vi "Generic command handler.vi"(8 "error in (no error)":errorcluster, 10 "Message in":refnum<class "GenericMessage.lvclass">=refnum, 11 "PockelCell in":refnum<class "PockelCell.lvclass">) -> (0 "error out":errorcluster, 2 "value":string, 3 "PockelCell out":refnum<class "PockelCell.lvclass">)   [LabVIEW 2012, in "PockelCell.lvclass"]
doc: "The generic_command_handler processes the command 'generic'. Commands which are not part of the predefined list of commands fall under the 'generic' command for special activity."
uses:
  PockelCell.lvclass
  <vilib>/Distrio/Murmex/Murmex/Murmex.lvclass
  Murmex/LabVIEW/Murmex/GenericMessage/GenericMessage.lvclass
panel:
  # "This method is called when the GENERIC\ntrigger is sent. \n\nOverride this method when your component needs to\nrespond to this trigger. \n\nCall parent for proper implementation"
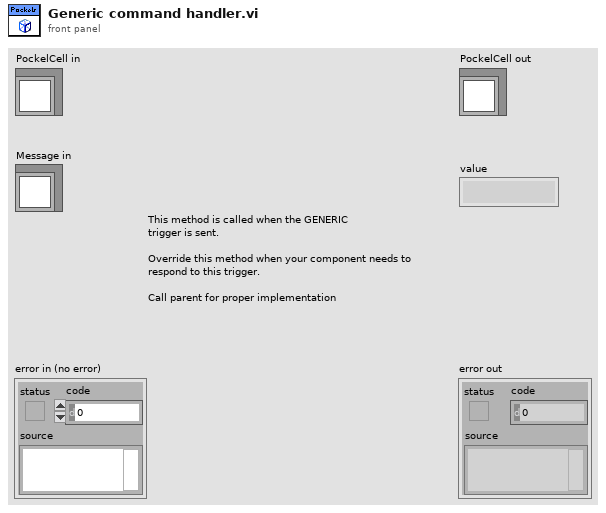
[diagram p1: front panel]
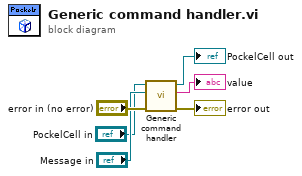
[diagram p0: block diagram]
diagram:
  n1 = call-parent "Generic command handler.vi"("error in (no error)"="error in (no error)", "Message in"="Message in", "Murmex in"="PockelCell in") -> ("error out"=→"error out":errorcluster, "value"=→"value":string, "Murmex out"=→"PockelCell out":refnum<class "PockelCell.lvclass">)  [unwired: 6 in]
